vi "v0.2_pto_desacelerar_http.vi"(7 "tiempo_ms":i32, 8 "error_in":errorcluster, 9 "FQ_Inicio":u32, 10 "FQ_Final":u32, 11 "mbed.lvclass IN":refnum<class "mbed.lvclass">) -> (0 "error out":errorcluster, 2 "FQ_salida":u32, 3 "mbed.lvclass OUT":refnum<class "mbed.lvclass">)   [LabVIEW 2011]
doc: "<B>Acelerar mediante PTO</B>\n\nEste VI se utiliza para decrementar la <B>frecuencia</B> del tren de pulsos. Envia un nuevo comando cada 1ms hasta alcanzar la frecuencia deseada."
uses:
  mbed/Transport Mechanisms/mbed/mbed.lvclass
  <vilib>/Platform/TimedLoop/XDataNode/timing_clust.ctl
  <vilib>/Platform/TimedLoop/XDataNode/nitl_modes.ctl
  <vilib>/Platform/TimedLoop/XDataNode/wakeup.ctl
  <vilib>/Platform/TimedLoop/XDataNode/XDataNode.xnode
  <vilib>/Platform/TimedLoop/XDataNode/XDNodeRunTimeDep.lvlib
panel:
  # "FUNCION ACELERACIÓN PARA LA FRECUENCIA DE SALIDA"
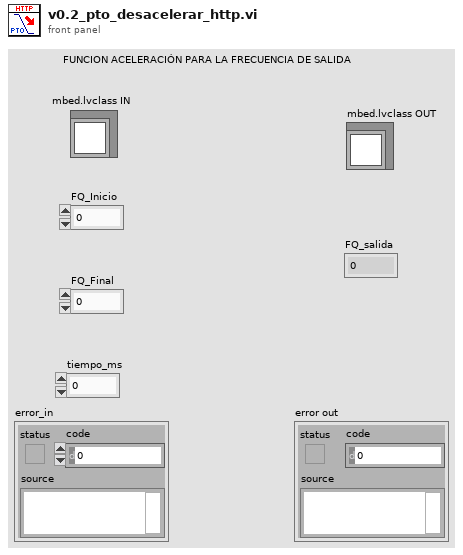
[diagram p1: front panel]
types:
  T1 = typedef "XDNodeRunTimeDep.lvlib/timing_clust.ctl" = cluster{"Expected End [f-1]":u64, "Actual End [f-1]":u64, "Finished Late? [f-1]":bool, "Expected End [i-1]":u64, "Actual End [i-1]":u64, "Finished Late? [i-1]":bool, "Expected Start [i]":u64, "Actual Start [i]":u64, "Expected Start [f]":u64, "Actual Start [f]":u64, "Source Name":string, "Structure Name":string, "Period":i64, "Deadline":i64, "Offset":i64, "Start":i64, "Priority":i32, "Timeout":i32, "Mode":T2, "Wakeup Reason":T3, "Error":errorcluster, "Source Type":string, "Secondary Source Type":string, "Global End Time":u64, "Global Start Time":u64, "Frame Duration":u64, "Iteration Duration":u64, "Assigned CPU":i32, "I/O Scan Engine Mode":u32}
  T2 = typedef "XDNodeRunTimeDep.lvlib/nitl_modes.ctl" = enum32{"No Change", "Process missed periods, maintain original phase", "Discard missed periods, maintain original phase", "Process missed periods, ignore original phase", "Discard missed periods, ignore original phase"}
  T3 = typedef "XDNodeRunTimeDep.lvlib/wakeup.ctl" = enum32{"Normal", "Aborted", "Asynchronous wakeup", "Timing source error", "Timed loop error", "Timeout"}
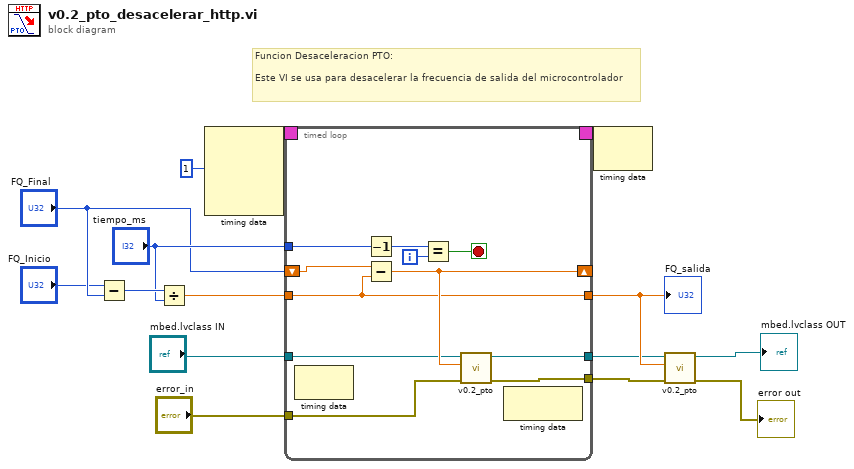
[diagram p0: block diagram]
diagram:
  # "Funcion Desaceleracion PTO:\n\nEste VI se usa para desacelerar la frecuencia de salida del microcontrolador"
  n1 = Subtract(x="FQ_Inicio", y="FQ_Final") -> (x-y=w15:u32)
  n2 = Divide(x=w15, y="tiempo_ms") -> (x/y=w10:dbl)
  n3 = node-c288(i64 1 ("Period")) -> (w14:T1)  [unwired: 3 in]
  n4 = timed-loop {
    timing: w14 -> [_]
    timing-out: [_] -> w13
    tunnel: "tiempo_ms" -> [w24]
    shift-right: [w22] -> _
    shift-left: "FQ_Final" -> [w20]
    tunnel: w10 -> [w19]
    tunnel: [w19] -> w8
    tunnel: [w21] -> w9
    tunnel: "error_in" -> [w18]
    tunnel: "mbed.lvclass IN" -> [w17]
    tunnel: [w16] -> w1
    i -> [w26]
    stop <- w25 stop-if-true
    n5 = node-c288() -> ()  [unwired: 1 in, 1 out]
    n6 = Decrement(x=w24) -> (x-1=w23:i32)
    n7 = Subtract(x=w20, y=w19) -> (x-y=w22:dbl)
    n8 = Equal?(x=w23, y=w26) -> (x = y?=w25:bool)
    n9 = call "v0.2_pto.vi"("error in"=w18, "Frecuencia"=w22, "mbed.lvclass IN"=w17) -> ("error out"=w21:errorcluster, "mbed.lvclass OUT"=w16:refnum<class "mbed.lvclass">)  [unwired: 7 in]
    n10 = node-c288() -> ()  [unwired: 1 in, 1 out]
  }
  "FQ_salida" <- w8
  n11 = node-c288(w13) -> ()  [unwired: 1 out]
  n12 = call "v0.2_pto.vi"("error in"=w9, "Frecuencia"=w8, "mbed.lvclass IN"=w1) -> ("error out"=→"error out":errorcluster, "mbed.lvclass OUT"=→"mbed.lvclass OUT":refnum<class "mbed.lvclass">)  [unwired: 7 in]
